vi "ObtainBroadcastForRegistration.vi"(8 "error in (no error)":errorcluster) -> (0 "error out":errorcluster, 2 "FgenBroadcastEvents":T1)   [LabVIEW 2018, in "FgenShared.lvlib"]
uses:
  FgenShared.lvlib
  clBroadcastEvents.ctl
  clEventType.ctl
panel:
  # "Rename this for each module type"
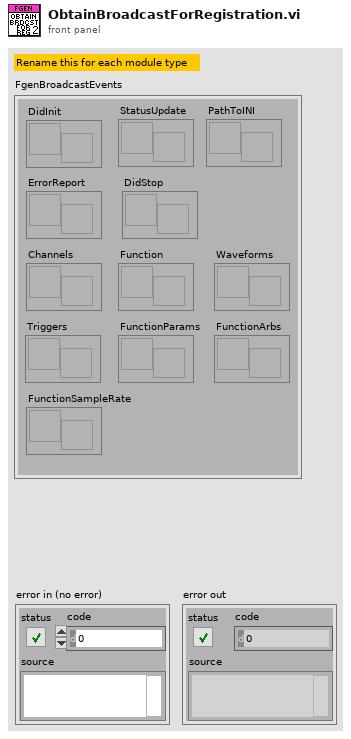
[diagram p1: front panel]
types:
  T1 = typedef "FgenShared.lvlib/clBroadcastEvents.ctl" = cluster{"DidInit":refnum<user-event>, "StatusUpdate":refnum<user-event>, "ErrorReport":refnum<user-event>, "DidStop":refnum<user-event>, "PathToINI":refnum<user-event>, "Channels":refnum<user-event>, "Function":refnum<user-event>, "Waveforms":refnum<user-event>, "Triggers":refnum<user-event>, "FunctionParams":refnum<user-event>, "FunctionArbs":refnum<user-event>, "FunctionSampleRate":refnum<user-event>}
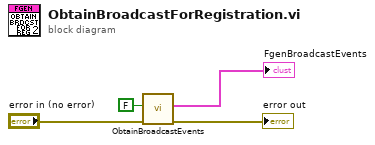
[diagram p0: block diagram]
diagram:
  n1 = call "ObtainBroadcastEvents.vi"("error in (no error)"="error in (no error)", "CreateNew? (F)"=FALSE) -> ("error out"=→"error out":errorcluster, "FgenBroadcastEvents"=→"FgenBroadcastEvents":T1)  [unwired: 8 in]
